vi "Building_Variants_after_Origin(101)-2.vi"(4 "[IN] Minimal Subtrack Length":i32, 5 "[IN] Subtrack":T1, 6 "[IN] Index in the Subtrack":i32, 7 "[IN] Indexes for Jumps":i32[](array[numeric]), 8 "error IN":errorcluster, 9 "[IN] Count of variants":i32, 10 "[IN] Subtracks":T3(array[cluster]), 11 "[IN] Still connected\ntracks in group":T2) -> (0 "error OUT":errorcluster, 1 "[OUT] Count of variants":i32, 2 "[OUT] Subtracks":T3(array[cluster]))   [LabVIEW 2013]
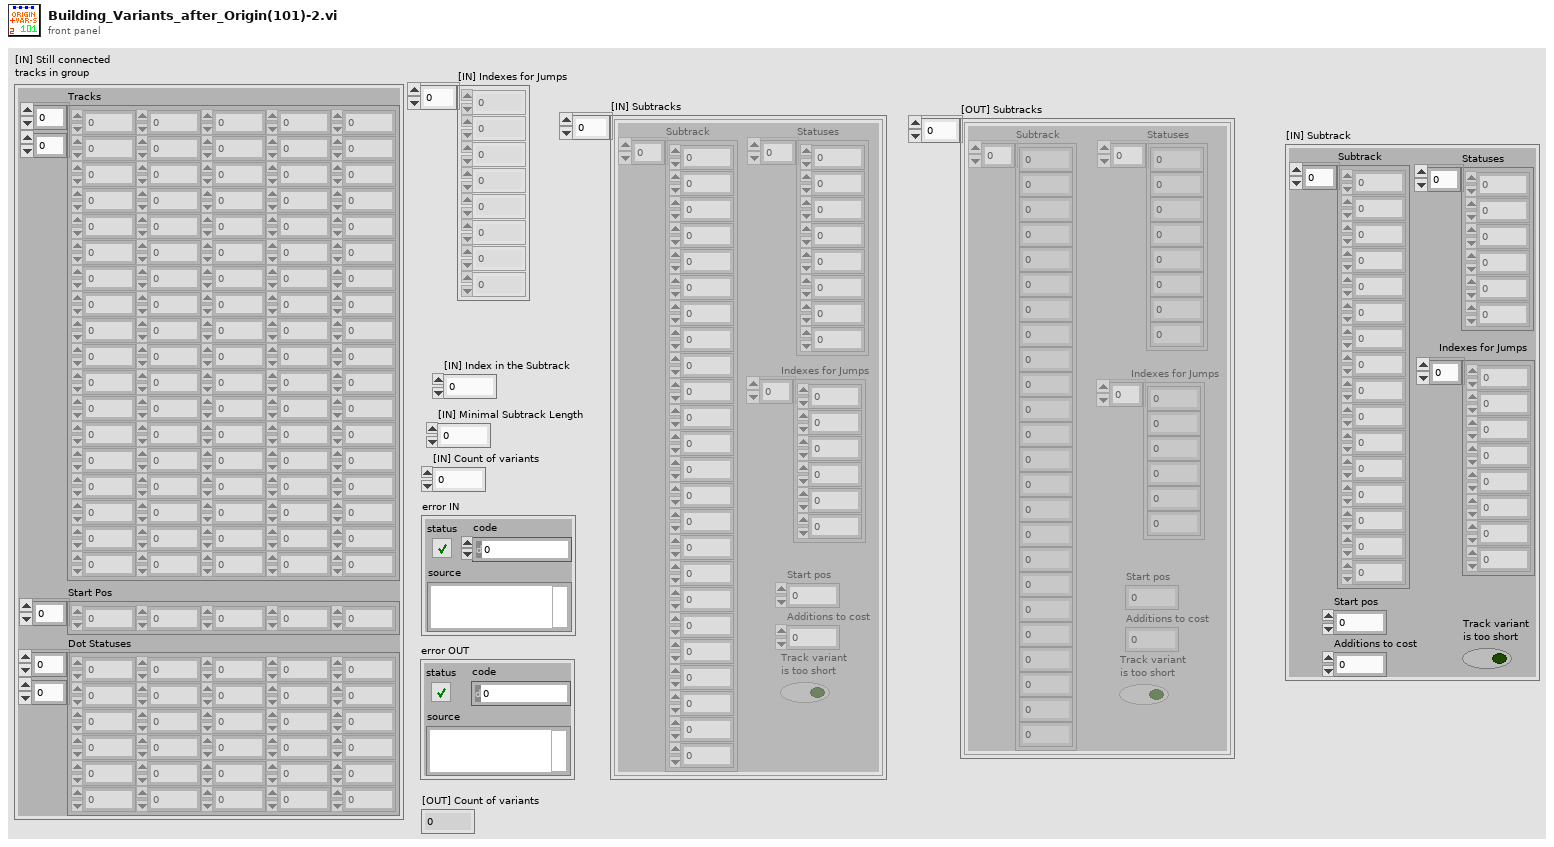
[diagram p1: front panel]
types:
  T1 = cluster{"Subtrack":dbl[], "Statuses":i16[], "Start pos":i32, "Additions to cost":i32, "Track variant \nis too short":bool, "Indexes for Jumps":i32[]}
  T2 = cluster{"Tracks":dbl[][], "Start Pos":i32[], "Dot Statuses":i16[][]}
  T3 = cluster{"Subtrack":dbl[], "Statuses":i16[], "Start pos":i32, "Additions to cost":i32, "Track variant \nis too short":bool, "Indexes for Jumps":i32[]}[]
  T4 = cluster{"Subtrack":dbl[], "Statuses":i16[], "Start pos":i32, "Additions to cost":i8, "Track variant \nis too short":bool, "Indexes for Jumps":i32[]}
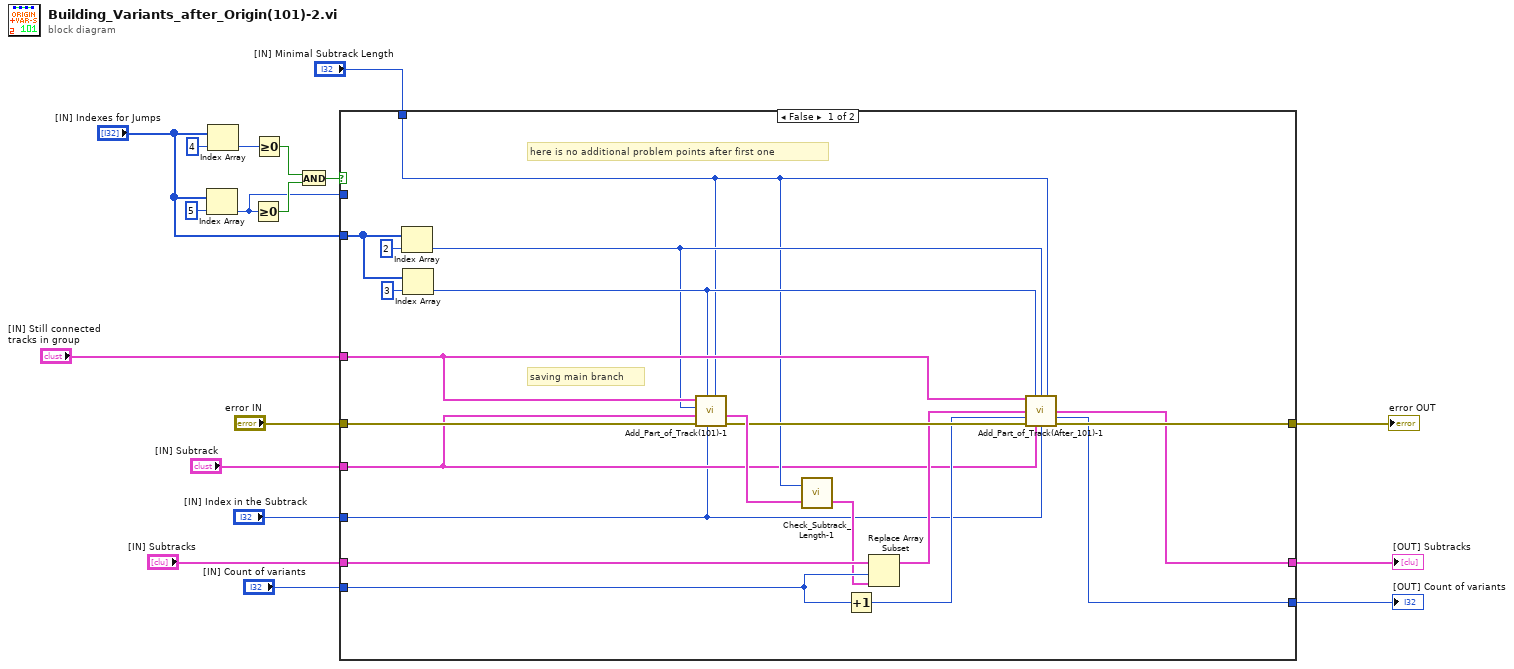
[diagram p0: block diagram]
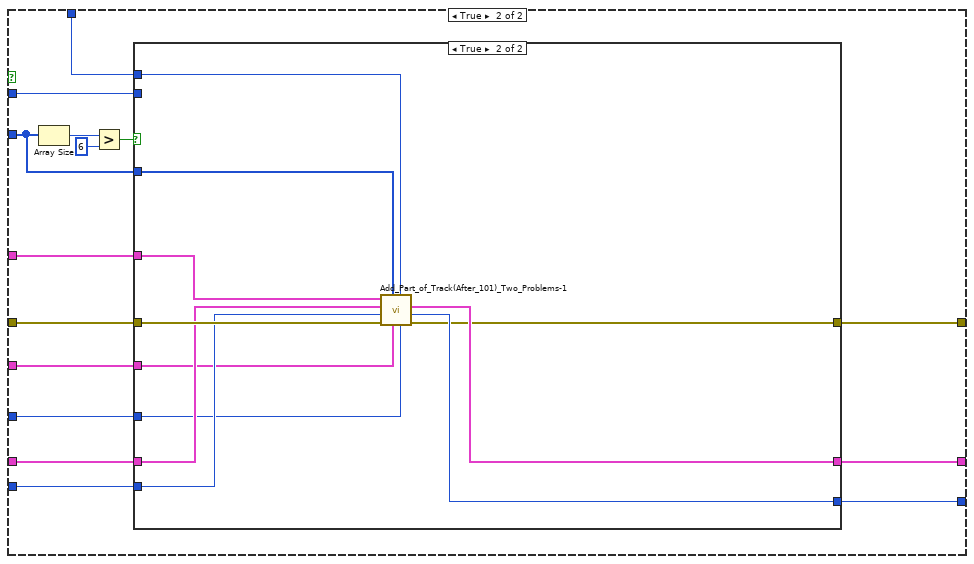
[diagram p2: hidden frame]
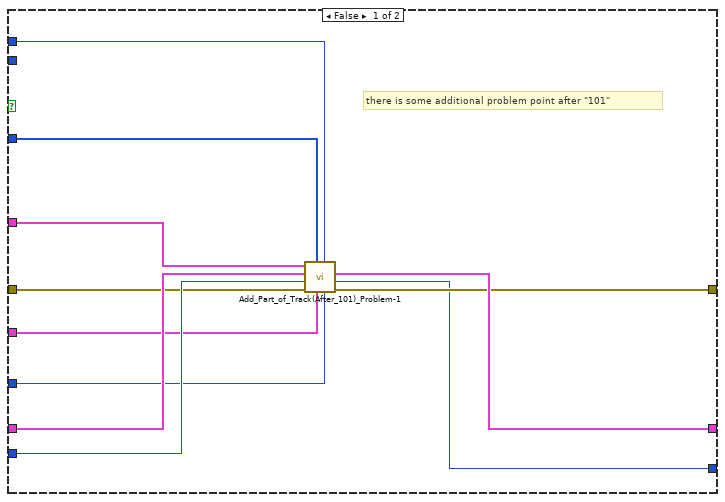
[diagram p3: hidden frame]
diagram:
  n1 = Index Array(array="[IN] Indexes for Jumps", index=5) -> (element=w12:i32)
  n2 = Index Array(array="[IN] Indexes for Jumps", index=4) -> (element=w13:i32)
  n3 = Greater Or Equal To 0?(x=w12) -> (x >= 0?=w15:bool)
  n4 = Greater Or Equal To 0?(x=w13) -> (x >= 0?=w16:bool)
  n5 = And(x=w16, y=w15) -> (x .and. y?=w14:bool)
  n6 = case shown="False" w14 {
    tunnel: w12 -> [_ w49]
    tunnel: "[IN] Indexes for Jumps" -> [w36 w42]
    tunnel: "[IN] Still connected\ntracks in group" -> [w29 w48]
    tunnel: "[IN] Subtrack" -> [w23 w50]
    tunnel: "error IN" -> [w33 w47]
    tunnel: "[IN] Index in the Subtrack" -> [w22 w45]
    tunnel: "[IN] Minimal Subtrack Length" -> [w26 w46]
    tunnel: "[IN] Subtracks" -> [w35 w44]
    tunnel: "[IN] Count of variants" -> [w34 w43]
    tunnel: [w20 w41] -> w2
    tunnel: [w19 w40] -> w1
    tunnel: [w21 w39] -> w3
    frame False {
      # "here is no additional problem points after first one"
      # "saving main branch"
      n7 = Index Array(array=w36, index=2) -> (element=w27:i32)
      n8 = Index Array(array=w36, index=3) -> (element=w28:i32)
      n9 = call "Add_Part_of_Track(101)-1.vi"("[IN] Minimal Sub\ntrack Length"=w26, "[IN] Index in subtrack"=w22, "[IN] # of subtrack conta\nining problem point"=w28, "error IN"=w33, "[IN] Subtrack"=w23, "[IN] Index of problem\npoint inside subtrack"=w27, "[IN] Still connected\ntracks in group"=w29) -> ("error OUT"=w30:errorcluster, "[OUT] Subtrack"=w32:T1)  [unwired: 2 in, 1 out]
      n10 = call "Check_Subtrack_Length-1.vi"("[IN] Subtrack"=w32, "[IN] Minimal Sub\ntrack Length"=w26) -> ("[OUT] Subtrack"=w31:T4)  [unwired: 1 in]
      n11 = Increment(x=w34) -> (x+1=w24:i32)
      n12 = Replace Array Subset(array=w35, new element=w31, index=w34) -> (w25:T3)
      n13 = call "Add_Part_of_Track(After_101)-1.vi"("[IN] Still connected\ntracks in group"=w29, "[IN] # of subtrack conta\nining problem point"=w28, "[IN] Index of problem\npoint inside subtrack"=w27, "[IN] Minimal Sub\ntrack Length"=w26, "[IN] Subtracks"=w25, "[IN] Count of variants"=w24, "error IN"=w30, "[IN] Subtrack"=w23, "[IN] Index in subtrack"=w22) -> ("[OUT] Subtracks"=w20:T3, "[OUT] Count of variants"=w19:i32, "error OUT"=w21:errorcluster)  [unwired: 4 in]
    }
    frame True {
      n14 = Array Size(array=w42) -> (size(s)=w53:i32)
      n15 = Greater?(x=w53, y=6) -> (0:w51:bool)
      n16 = case shown="True" w51 {
        tunnel: w50 -> [w58 w69]
        tunnel: w49 -> [_ _]
        tunnel: w48 -> [w61 w74]
        tunnel: w47 -> [w62 w75]
        tunnel: w46 -> [w59 w72]
        tunnel: w45 -> [w57 w68]
        tunnel: w44 -> [w64 w71]
        tunnel: w43 -> [w63 w70]
        tunnel: [w56 w67] -> w41
        tunnel: [w54 w66] -> w40
        tunnel: w42 -> [w60 w73]
        tunnel: [w55 w65] -> w39
        frame False {
          # "there is some additional problem point after \"101\""
          n17 = call "Add_Part_of_Track(After_101)_Problem-1.vi"("[IN] Index in subtrack"=w57, "[IN] Minimal Sub\ntrack Length"=w59, "[IN] Subtrack"=w58, "[IN] Indexes for Jumps"=w60, "error IN"=w62, "[IN] Count of variants"=w63, "[IN] Subtracks"=w64, "[IN] Still connected\ntracks in group"=w61) -> ("error OUT"=w55:errorcluster, "[OUT] Count of variants"=w54:i32, "[OUT] Subtracks"=w56:T3)  [unwired: 1 in]
        }
        frame True {
          n18 = call "Add_Part_of_Track(After_101)_Two_Problems-1.vi"("[IN] Index in subtrack"=w68, "[IN] Minimal Sub\ntrack Length"=w72, "[IN] Subtrack"=w69, "[IN] Indexes for Jumps"=w73, "error IN"=w75, "[IN] Count of variants"=w70, "[IN] Subtracks"=w71, "[IN] Still connected\ntracks in group"=w74) -> ("error OUT"=w65:errorcluster, "[OUT] Count of variants"=w66:i32, "[OUT] Subtracks"=w67:T3)  [unwired: 1 in]
        }
      }
    }
  }
  "[OUT] Subtracks" <- w2
  "error OUT" <- w3
  "[OUT] Count of variants" <- w1
